vi "TextFit_Extract Bitmap and size.vi"(6 "Last Character":bool, 8 "Error":errorcluster, 11 "Character Cluster":T1) -> (0 "Error Out":errorcluster, 3 "BitMap Out":T4, 5 "Size Out":i32)   [LabVIEW 2014]
doc: "Gets the BitMap array from the font array based on the character cluster"
uses:
  Controls/Array/Array Bool Char Bits Wide.ctl
  Controls/Cluster/Cluster_Character Size and Priority Data.ctl
  Controls/String_Picture/String Char Normal.ctl
  Controls/Enum/ENUM_Font Size Select.ctl
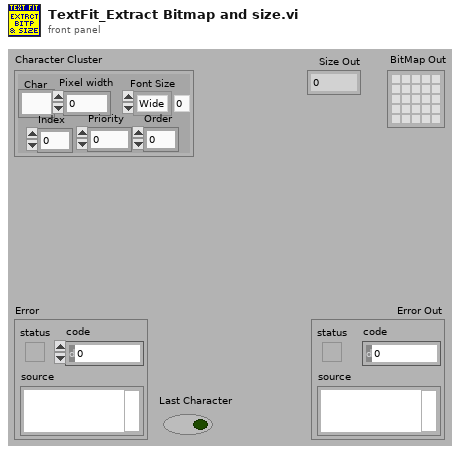
[diagram p1: front panel]
types:
  T1 = typedef "Cluster_Character Size and Priority Data.ctl" = cluster{"Char":T2, "Font Size":T3, "Pixel width":i32, "Priority":i32, "Order":i32, "Index":i32}
  T2 = typedef "String Char Normal.ctl" = string
  T3 = typedef "ENUM_Font Size Select.ctl" = enum16{"Wide", "Med", "Thin"}
  T4 = typedef "Array Bool Char Bits Wide.ctl" = bool[][]
  T5 = typedef "Cluster_Font Data.ctl" = cluster{"Font List Out":T6[], "Char Array":T2[], "Seperator Index":i32}
  T6 = typedef "Cluster_Character Data.ctl" = cluster{"Char":T2, "Wide":T4, "Med":T7, "Thin":T8, "Priority":i32}
  T7 = typedef "Array Bool Char Bits Med.ctl" = bool[][]
  T8 = typedef "Array Bool Char Bits Thin.ctl" = bool[][]
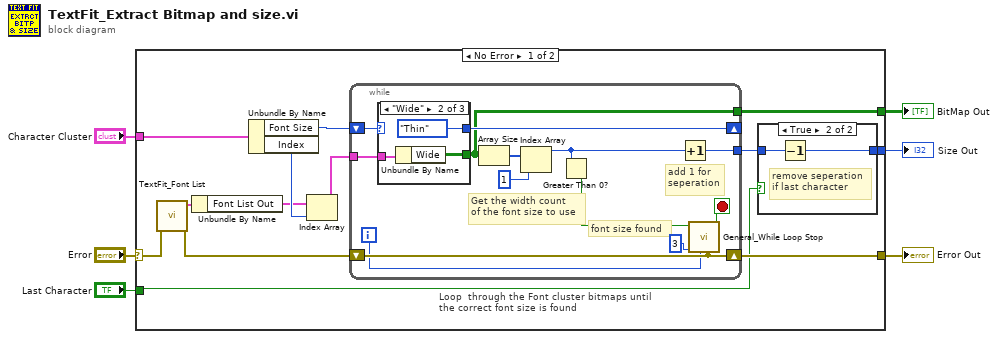
[diagram p0: block diagram]
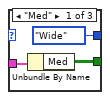
[diagram p3: hidden frame]
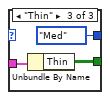
[diagram p4: hidden frame]
diagram:
  n1 = case shown="No Error" "Error" {
    selector: "Error" -> [w7 w45]
    tunnel: [w19 _] -> w6
    tunnel: [w18 w45] -> w5
    tunnel: "Last Character" -> [w17 _]
    tunnel: [w15 _] -> w3
    tunnel: "Character Cluster" -> [w14 _]
    frame No Error {
      n2 = call "TextFit_Font List.vi"("Error In"=w7) -> ("Error Out"=w8:errorcluster, "Font Cluster Out"=w10:T5)  [unwired: 9 in]
      n3 = Unbundle By Name(w10) -> ("Font List Out"=w9:T6[])
      n4 = Unbundle By Name(w14) -> ("Font Size"=w13:T3, "Index"=w12:i32)
      n5 = Index Array(array=w9, index=w12) -> (element=w11:T6)
      n6 = while "Loop  through the Font cluster bitmaps until the correct font size is found" {
        tunnel: w11 -> [w35]
        tunnel: [w28] -> w16
        shift-right: [w31] -> _
        shift-left: w13 -> [w29]
        shift-right: [w30] -> w18
        shift-left: w8 -> [w30]
        tunnel: [w27] -> w19
        i -> [w24]
        stop <- w26 stop-if-true
        # "add 1 for\nseperation"
        # "font size found"
        # "Get the width count\nof the font size to use"
        n7 = case shown="\"Wide\"" w29 {
          tunnel: w35 -> [w38 w41 w44]
          tunnel: [w37 w40 w43] -> w27
          tunnel: [ENUM_Font_Size_Select."Wide" ("Font Size Select") ENUM_Font_Size_Select."Thin" ("Font Size Select") ENUM_Font_Size_Select."Med" ("Font Size Select")] -> w31
          frame "Med" {
            n8 = Unbundle By Name(w38) -> ("Med"=w37:T7)
          }
          frame "Wide" {
            n9 = Unbundle By Name(w41) -> ("Wide"=w40:T4)
          }
          frame "Thin" {
            n10 = Unbundle By Name(w44) -> ("Thin"=w43:T8)
          }
        }
        n11 = Array Size(array=w27) -> (size(s)=w34:i32[])
        n12 = Index Array(array=w34, index=1) -> (element=w32:i32)
        n13 = Greater Than 0?(x=w32) -> (x > 0?=w25:bool)
        n14 = Increment(x=w32) -> (x+1=w28:i32)
        n15 = call "General_While Loop Stop.vi"("Error In"=w30, "Index In"=w24, "Array Size In"=3, "Stop 1 In"=w25) -> ("Stop Out1"=w26:bool)  [unwired: 3 in, 3 out]
      }
      n16 = case shown="True" w17 {
        tunnel: w16 -> [w20 w22]
        tunnel: [w20 w21] -> w15
        frame False {
        }
        frame True {
          # "remove seperation\nif last character"
          n17 = Decrement(x=w22) -> (x-1=w21:i32)
        }
      }
    }
    frame Error {
    }
  }
  "BitMap Out" <- w6
  "Error Out" <- w5
  "Size Out" <- w3
